vi "Build Tree Data Type.vi"(4 "Tag Blacklist":i8[](array[numeric]), 6 "Show IDs (True)":bool=TRUE, 7 "Test ID":string, 8 "error in (no error)":errorcluster, 11 "Test Executive Ref":refnum<data-value>) -> (0 "error out":errorcluster, 2 "Tree Data":T1(array[cluster]), 3 "Test Executive Ref out":refnum<data-value>)   [LabVIEW 2019, in "Test Executive.lvlib" / "TestExecutive Ref.lvclass"]
uses:
  <vilib>/gpm_packages/@cs/test-executive/Source/Test Executive/TestExecutive Ref/TestExecutive Ref.lvclass
  <vilib>/gpm_packages/@cs/test-executive/Source/Test Executive/ITestExecutive/ITest Executive.lvclass
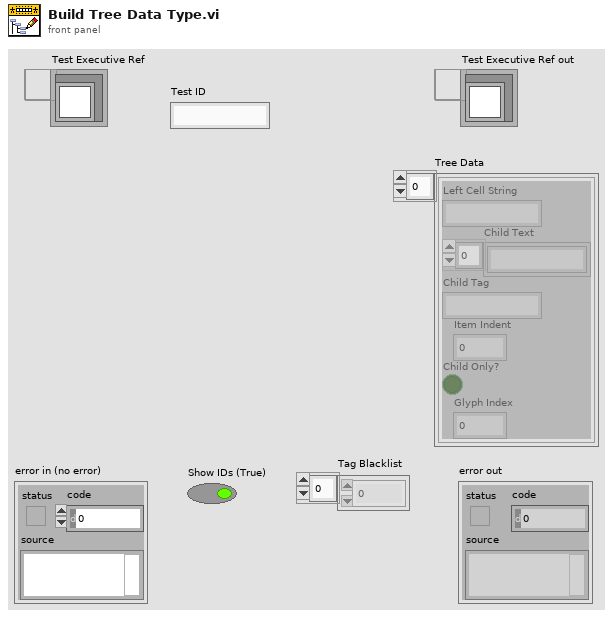
[diagram p1: front panel]
types:
  T1 = cluster{"Left Cell String":string, "Child Text":string[], "Child Tag":string, "Item Indent":i32, "Child Only?":bool, "Glyph Index":i32}[]
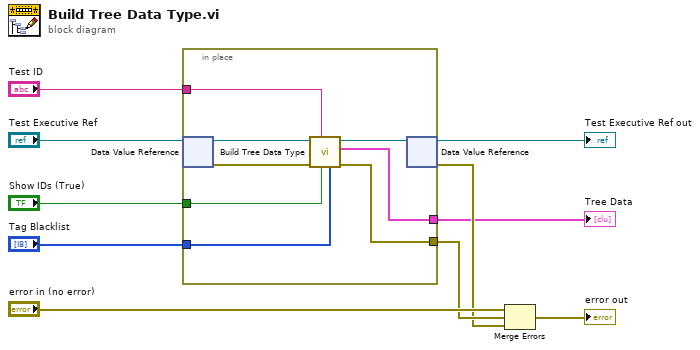
[diagram p0: block diagram]
diagram:
  n1 = in-place {
    in-place-border: "Test ID" -> [w16]
    in-place-border: [w14] -> w6
    in-place-border: "Show IDs (True)" -> [w13]
    in-place-border: [w12] -> w2
    in-place-border: "Tag Blacklist" -> [w11]
    n2 = in-place-dvr #1("Test Executive Ref") -> (w18:refnum<class "ITest Executive.lvclass">, w15:errorcluster)
    n3 = call-dynamic "Build Tree Data Type.vi"("Tag Blacklist"=w11, "Show IDs (True)"=w13, "Test ID"=w16, "error in (no error)"=w15, "ITest Executive in"=w18) -> ("error out"=w14:errorcluster, "Tree Data"=w12:T1, "ITest Executive out"=w17:refnum<class "ITest Executive.lvclass">)  [unwired: 4 in]
    n4 = in-place-dvr #1(w17) -> (→"Test Executive Ref out":refnum<data-value>, w5:errorcluster)
  }
  "Tree Data" <- w2
  n5 = Merge Errors("error in (no error)", w6, w5) -> (→"error out":errorcluster)
